vi "Apply Step Configuration.vi"(8 "error in (no error)":errorcluster, 9 "Measurement Actor.lvlib:Step Configuration.lvclass":refnum<class "Step Configuration.lvclass">, 10 "Measurement Name":string, 11 "Controller in":refnum<class "Controller.lvclass">) -> (0 "error out":errorcluster, 3 "Controller out":refnum<class "Controller.lvclass">)   [LabVIEW 2026, in "Controller Actor.lvlib" / "Controller.lvclass"]
uses:
  Controller.lvclass
  Measurement Actor/Configuration/Step Configuration.lvclass
  Measurement Actor/Measurement.lvclass/Measurement.ctl
  Controller.lvclass/Controller.ctl
  Measurement Actor/Measurement.lvclass
panel:
  out "replaced":bool
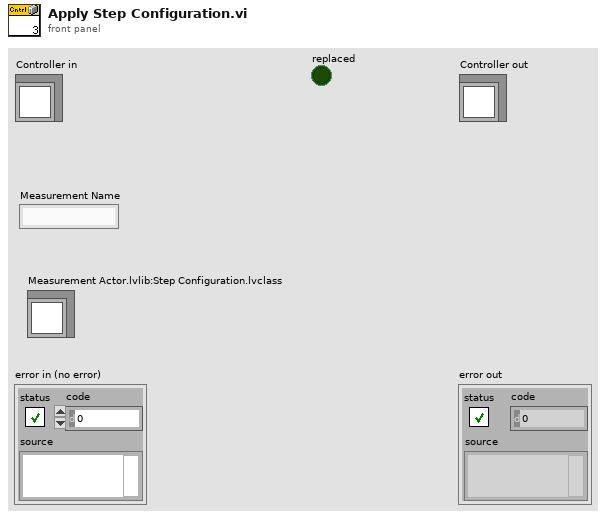
[diagram p1: front panel]
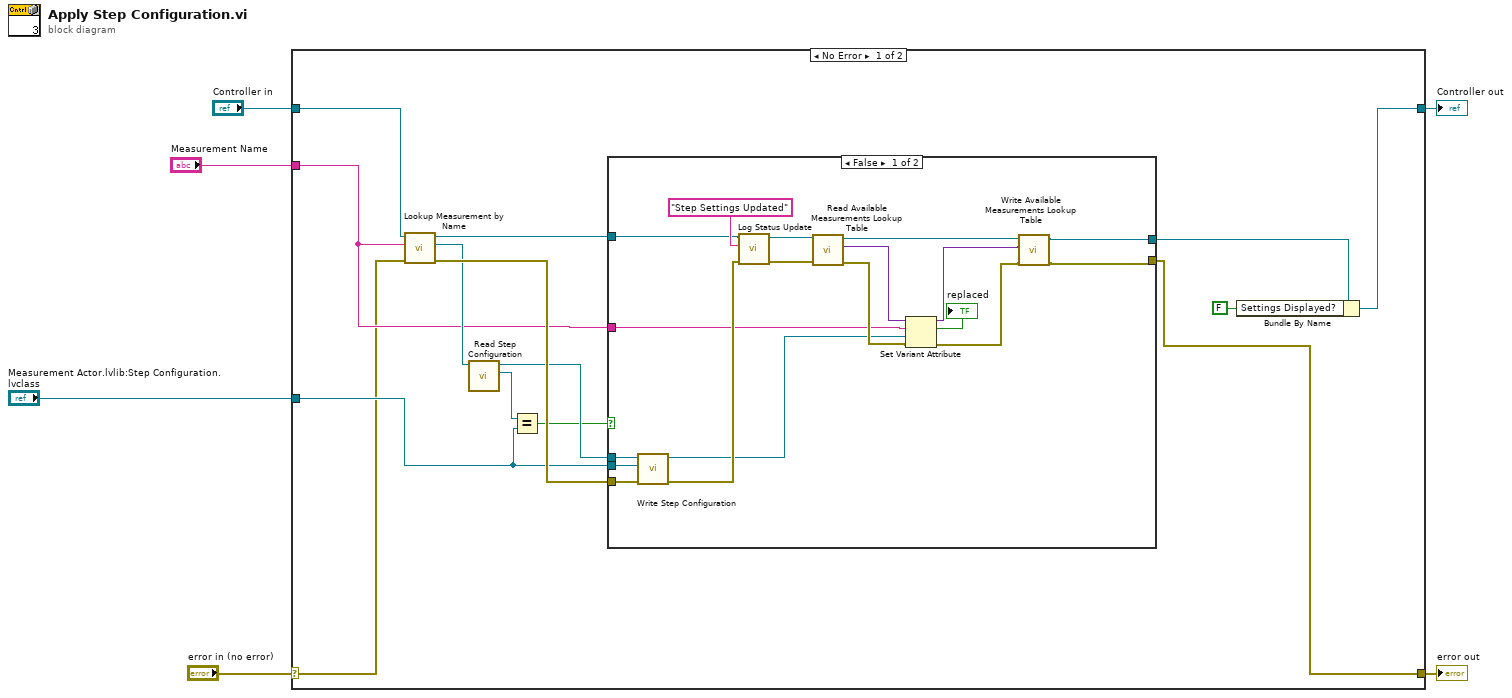
[diagram p0: block diagram]
diagram:
  n1 = case shown="No Error" "error in (no error)" {
    selector: "error in (no error)" -> [w8 w42]
    tunnel: [w7 w42] -> w5
    tunnel: [w9 w41] -> w3
    tunnel: "Controller in" -> [w11 w41]
    tunnel: "Measurement Actor.lvlib:Step Configuration.lvclass" -> [w12 _]
    tunnel: "Measurement Name" -> [w10 _]
    frame No Error {
      n2 = call "Lookup Measurement by Name.vi"("error in (no error)"=w8, "Measurement Name"=w10, "Controller in"=w11) -> ("error out"=w20:errorcluster, "Measurement.lvclass"=w18:refnum<class "Measurement.lvclass">, "Controller out"=w15:refnum<class "Controller.lvclass">)  [unwired: 5 in, 1 out]
      n3 = call "Read Step Configuration.vi"("Measurement in"=w18) -> ("Measurement Actor.lvlib:Step Configuration.lvclass"=w16:refnum<class "Step Configuration.lvclass">, "Measurement out"=w17:refnum<class "Measurement.lvclass">)  [unwired: 8 in, 1 out]
      n4 = Equal?(x=w16, y=w12) -> (x = y?=w14:bool)
      n5 = case shown="False" w14 {
        tunnel: w20 -> [w38 w40]
        tunnel: w17 -> [w37 _]
        tunnel: w12 -> [w36 _]
        tunnel: w15 -> [w34 w39]
        tunnel: w10 -> [w28 _]
        tunnel: [w21 w39] -> w13
        tunnel: [w24 w40] -> w7
        frame False {
          n6 = call "Write Step Configuration.vi"("error in (no error)"=w38, "Measurement Actor.lvlib:Step Configuration.lvclass"=w36, "Measurement in"=w37) -> ("error out"=w33:errorcluster, "Measurement out"=w27:refnum<class "Measurement.lvclass">)  [unwired: 7 in]
          n7 = call-dynamic "Log Status Update.vi"("error in (no error)"=w33, "String"="Step Settings Updated", "Controller in"=w34) -> ("error out"=w30:errorcluster, "Controller out"=w29:refnum<class "Controller.lvclass">)  [unwired: 7 in]
          n8 = call "Read Available Measurements Lookup Table.vi"("error in (no error)"=w30, "Controller in"=w29) -> ("error out"=w32:errorcluster, "Available Measurements Lookup Table"=w31:variant, "Controller out"=w22:refnum<class "Controller.lvclass">)  [unwired: 7 in]
          n9 = Set Variant Attribute(Variant=w31, name=w28, value=w27, error in=w32) -> (Variant out=w23:variant, replaced=→"replaced":bool, error out=w25:errorcluster)
          n10 = call "Write Available Measurements Lookup Table.vi"("error in (no error)"=w25, "Available Measurements Lookup Table"=w23, "Controller in"=w22) -> ("error out"=w24:errorcluster, "Controller out"=w21:refnum<class "Controller.lvclass">)  [unwired: 7 in]
        }
        frame True {
        }
      }
      n11 = Bundle By Name(cluster=w13, "Settings Displayed?"=FALSE) -> (w9:refnum<class "Controller.lvclass">)
    }
    frame Error {
    }
  }
  "error out" <- w5
  "Controller out" <- w3
